vi "SalvaImpostazioni_OUTPUT.vi"(10 "banco":i32, 11 "Array Misure Output":dbl[](array[numeric])) -> ()   [LabVIEW 2019]
uses:
  TypeDef/ClusterCaratteristicheMisura_OUTPUT.ctl
panel:
  in  "Array ClusterCaratteristicheMisura":T1[](array[typedef])
  in  "Salva Impostazioni":bool
  out "Numero di misure":i32
  in  "Carica Impostazioni":bool
  in  "Stop":bool
  # "RISERVATO AD USO\nINTESYS"
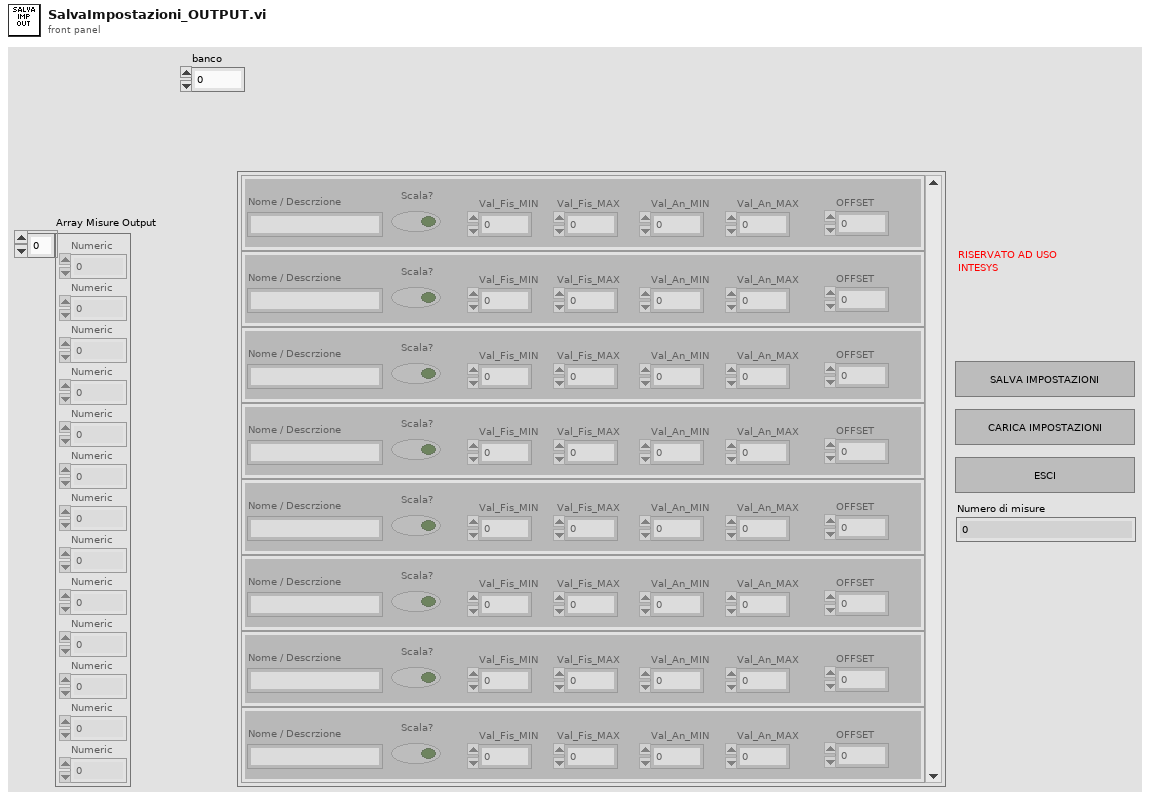
[diagram p1: front panel]
types:
  T1 = typedef "ClusterCaratteristicheMisura_OUTPUT.ctl" = cluster{"Nome / Descrzione":string, "Scala?":bool, "Val_Fis_MIN":dbl, "Val_Fis_MAX":dbl, "Val_An_MIN":dbl, "Val_An_MAX":dbl, "OFFSET":dbl}
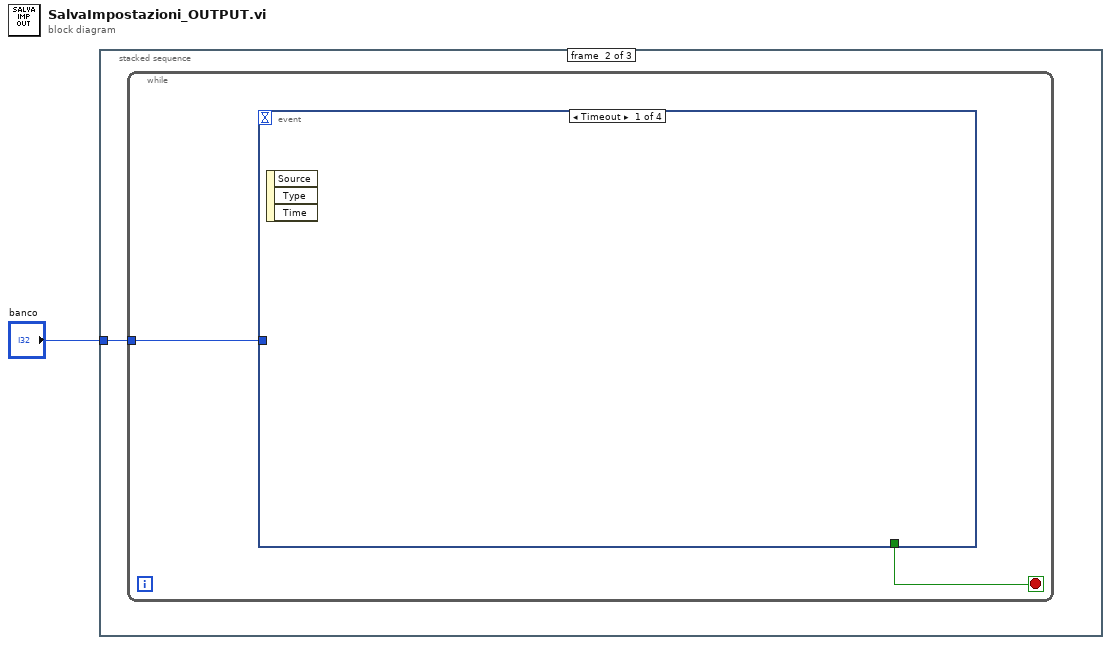
[diagram p0: block diagram]
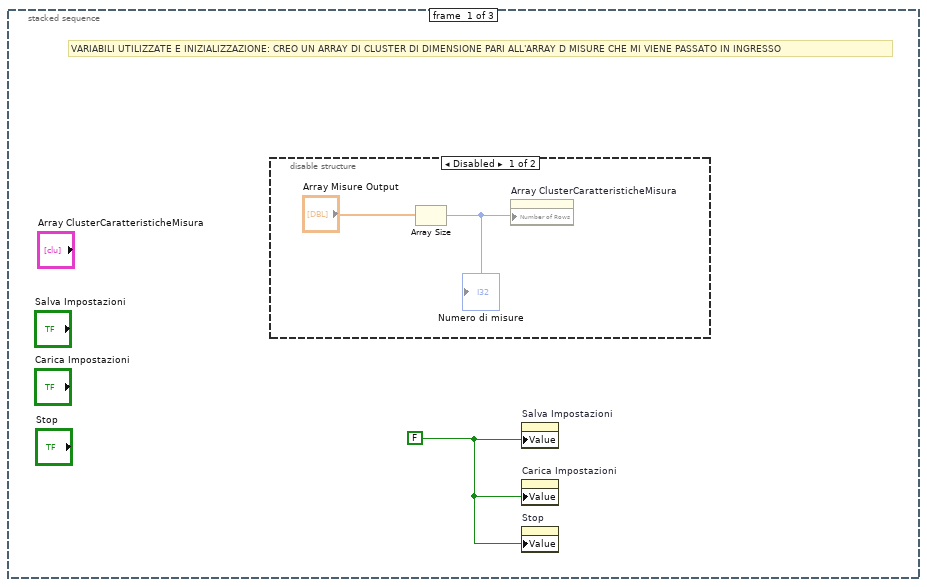
[diagram p2: hidden frame]
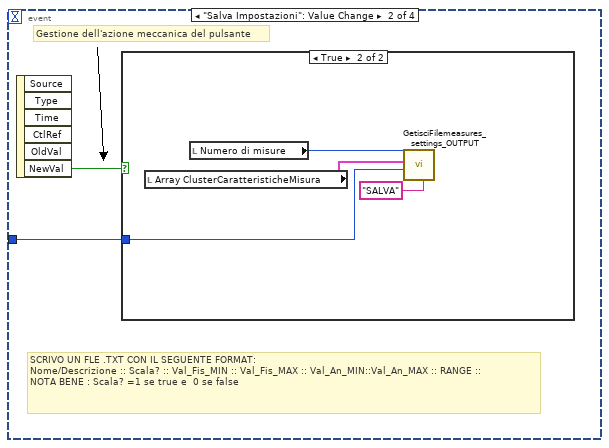
[diagram p4: hidden frame]
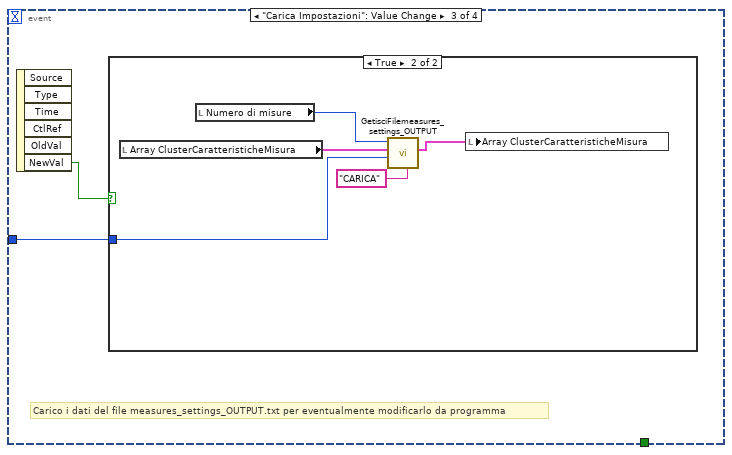
[diagram p6: hidden frame]
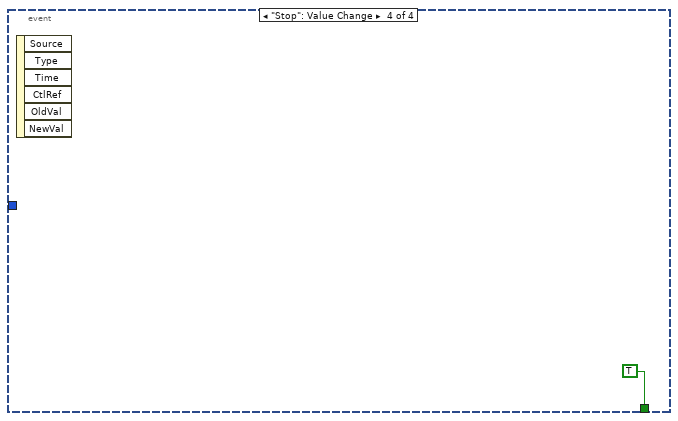
[diagram p8: hidden frame]
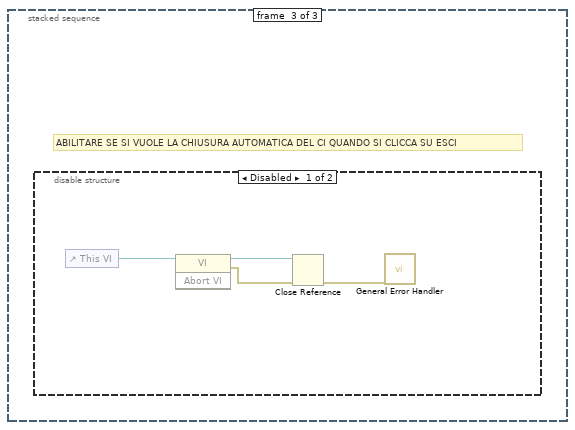
[diagram p9: hidden frame]
diagram:
  n1 = stacked-sequence {
    tunnel: "banco" -> [_ w5 _]
    frame #0 {
      w2 = FALSE ("Salva Impostazioni")
      # "VARIABILI UTILIZZATE E INIZIALIZZAZIONE: CREO UN ARRAY DI CLUSTER DI DIMENSIONE PARI ALL'ARRAY D MISURE CHE MI VIENE PASSATO IN INGRESSO"
      n2 = disable-structure shown="Disabled" {
        frame Disabled {
          n3 = Array Size(array="Array Misure Output") -> (size(s)=w3:i32)
          "Numero di misure" <- w3
          n4 = property on="Array ClusterCaratteristicheMisura" class="Arr (strict)"("Number of Rows"=w3) -> ()  [unwired: 2 in, 2 out]
        }
        frame Enabled {
        }
      }
      n5 = property on="Salva Impostazioni" class="Bool (strict)"("Value"=w2) -> ()  [unwired: 2 in, 2 out]
      n6 = property on="Carica Impostazioni" class="Bool (strict)"("Value"=w2) -> ()  [unwired: 2 in, 2 out]
      n7 = property on="Stop" class="Bool (strict)"("Value"=w2) -> ()  [unwired: 2 in, 2 out]
    }
    frame #1 {
      n8 = while {
        tunnel: w5 -> [w6]
        stop <- w7 stop-if-true
        n9 = event shown="[0] Timeout" {
          selector: _ -> [_ _ _ _]
          dyn-events: _ -> [_ _ _ _]
          timeout: _ -> [_ _ _ _]
          tunnel: [_ _ _ TRUE] -> w7
          tunnel: w6 -> [_ w8 w14 _]
          event Timeout {
            n10 = event-data() -> ()  [unwired: 1 in, 3 out]
          }
          event "Salva Impostazioni": Value Change {
            # "Gestione dell'azione meccanica del pulsante"
            # "SCRIVO UN FLE .TXT CON IL SEGUENTE FORMAT:\nNome/Descrizione :: Scala? :: Val_Fis_MIN :: Val_Fis_MAX :: Val_An_MIN::Val_An_MAX :: RANGE ::  \nNOTA BENE : Scala? =1 se true e  0 se false"
            n11 = event-data() -> ("NewVal"=w9:bool)  [unwired: 1 in, 5 out]
            n12 = case shown="True" w9 {
              tunnel: w8 -> [_ w10]
              frame False {
              }
              frame True {
                n13 = local read "Array ClusterCaratteristicheMisura"() -> (w12:T1[])
                n14 = local read "Numero di misure"() -> (w13:i32)
                n15 = call "GetisciFilemeasures_settings_OUTPUT.vi"("Azione"="SALVA", "banco"=w10, "Array ClusterCaratteristicheMisura IN"=w12, "Numero Misure"=w13) -> ()  [unwired: 7 in, 1 out]
              }
            }
          }
          event "Carica Impostazioni": Value Change {
            # "Carico i dati del file measures_settings_OUTPUT.txt per eventualmente modificarlo da programma"
            n16 = event-data() -> ("NewVal"=w15:bool)  [unwired: 1 in, 5 out]
            n17 = case shown="True" w15 {
              tunnel: w14 -> [_ w17]
              frame False {
              }
              frame True {
                n18 = local read "Array ClusterCaratteristicheMisura"() -> (w19:T1[])
                n19 = local read "Numero di misure"() -> (w18:i32)
                n20 = call "GetisciFilemeasures_settings_OUTPUT.vi"("Azione"="CARICA", "banco"=w17, "Array ClusterCaratteristicheMisura IN"=w19, "Numero Misure"=w18) -> ("Array ClusterCaratteristicheMisura OUT"=w16:T1[])  [unwired: 7 in]
                n21 = local write "Array ClusterCaratteristicheMisura"(w16) -> ()
              }
            }
          }
          event "Stop": Value Change {
            n22 = event-data() -> ()  [unwired: 1 in, 6 out]
          }
        }
      }
    }
    frame #2 {
      # "ABILITARE SE SI VUOLE LA CHIUSURA AUTOMATICA DEL CI QUANDO SI CLICCA SU ESCI"
      n23 = disable-structure shown="Disabled" {
        frame Disabled {
          n24 = control-ref of="This VI"() -> (w25:refnum<vi>)
          n25 = invoke class="VI" method="Abort VI"(reference=w25) -> (reference out=w24:refnum<vi>, error out=w22:errorcluster)  [unwired: 2 in, 1 out]
          n26 = Close Reference(reference=w24, error in (no error)=w22) -> (error out=w23:errorcluster)
          n27 = call <vilib>:"General Error Handler.vi"("error in (no error)"=w23) -> ()  [unwired: 10 in, 5 out]
        }
        frame Enabled {
        }
      }
    }
  }
